vi "A33ConfigureARB_py.vi"(8 "error in (no error)":errorcluster, 10 "Instrument":string="AG33600A_Gen1", 11 "socket in":refnum<class "zmq_socket.lvclass">) -> (0 "error out":errorcluster, 1 "Standalone":bool, 2 "resulting string":string, 3 "socket out":refnum<class "zmq_socket.lvclass">)   [LabVIEW 2022 SP3]
doc: "Selects the waveform shape, frequency, amplitude, offset, and phase for a standard waveform."
uses:
  <vilib>/addons/zeromq/zmq_socket.lvclass
panel:
  in  "F/SR/P? (0: Frequency)":i32(ring) items=["Frequency", "Sample rate", "Period"]
  in  "Advance mode (0: norm; 1:trig)":i32(ring) items=["Normal", "Triggered"]
  in  "Filter (0: OFF)":i32(ring) items=["OFF", "STEP", "NORM"]
  in  "ARB Number":i32=1
  in  "Phase (0 deg)":dbl format="%#_12g"
  in  "Freq/SRate/Period (1 Hz)":dbl=1.0 format="%#_12g"
  in  "DC Offset (0.0 V)":dbl format="%#_12g"
  in  "Amplitude (1.0 Vpp)":dbl=1.0 format="%#_12g"
  in  "Channel (1: Channel1)":i32(ring)=1 items=["Channel1"=1, "Channel2"=2]
  # "Positive # - selects wfm from volatile. Wfm must be loaded first.\nNegative - selects wfm loaded from non-vol memory, wfm must be first loaded into volatile from file!"
  # "Sometimes shows error message - it's ok, it's just\nphase sync command"
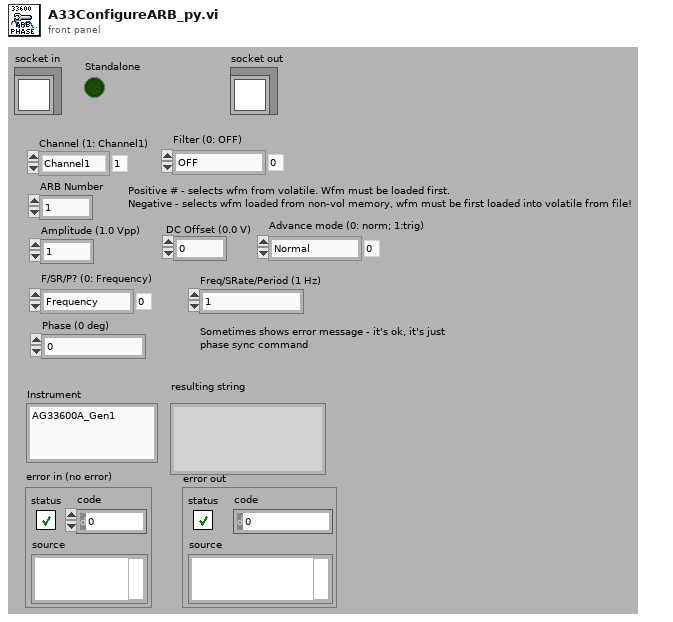
[diagram p1: front panel]
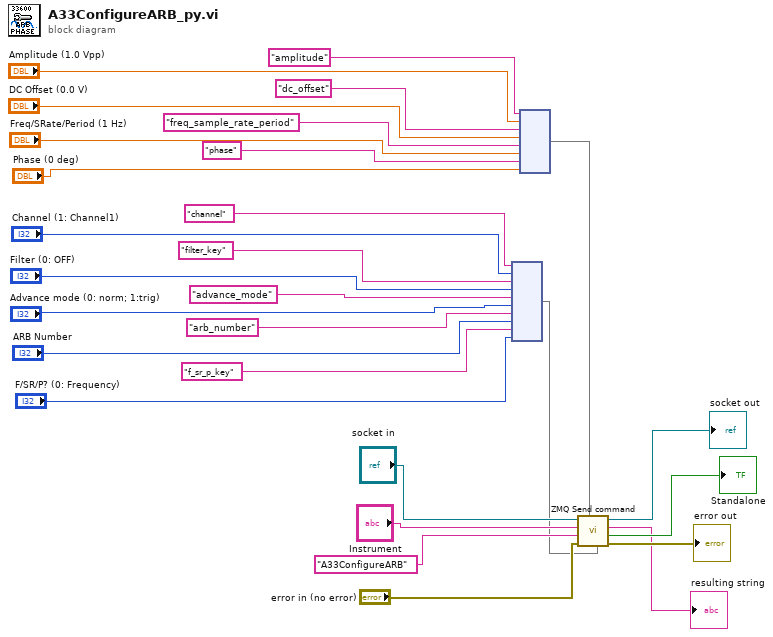
[diagram p0: block diagram]
diagram:
  n1 = node("channel" ("key"), "Channel (1: Channel1)", "filter_key" ("key"), "Filter (0: OFF)", "advance_mode" ("key"), "Advance mode (0: norm; 1:trig)", "arb_number" ("key"), "ARB Number", "f_sr_p_key" ("key"), "F/SR/P? (0: Frequency)") -> (w1:map{string, i32})
  n2 = node("amplitude" ("key"), "Amplitude (1.0 Vpp)", "dc_offset" ("key"), "DC Offset (0.0 V)", "freq_sample_rate_period" ("key"), "Freq/SRate/Period (1 Hz)", "phase" ("key"), "Phase (0 deg)") -> (w12:map{string, dbl})
  n3 = call "ZMQ Send command.vi"("Int args"=w1, "DBL args"=w12, "error in"="error in (no error)", "Command"="A33ConfigureARB", "Instrument"="Instrument", "socket in"="socket in") -> ("error out"=→"error out":errorcluster, "Standalone"=→"Standalone":bool, "Recieved message"=→"resulting string":string, "socket out"=→"socket out":refnum<class "zmq_socket.lvclass">)  [unwired: 2 in]
